vi "Pendulum get Msg Count.vi"(11 "instance":i32) -> (3 "function return":u32)   [LabVIEW 2024, in "pendulumApp.lvlib"]
doc: "OOTB_API unsigned long long Pendulum_getMsgCount(int instance);"
uses:
  pendulumApp.lvlib
  pendulumApp.dll
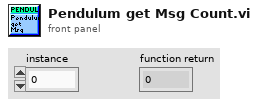
[diagram p1: front panel]
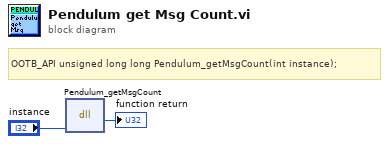
[diagram p0: block diagram]
diagram:
  # "OOTB_API\tunsigned long long Pendulum_getMsgCount(int instance);"
  n1 = dll-call lib="C:/Users/scer/OneDrive - University of Florida/eml4314c/eml4314cFA25/Resources/FA25_dev_version2/SADI_Pendulum_lib/pendulumApp.*" fn="Pendulum_getMsgCount"("instance"="instance") -> (→"function return":u32)  [unwired: 4 in, 2 out]
